vi "__GetDSA_35670A.vi"(11 "DSA_mes":T1={"GPIB_DSA"="11", "Startfrq(Hz)"=0.0, "Stopfrq(Hz)"=800.0, "Range(Vpk)"=1.0, "average"=4}) -> (0 "電圧":dbl[](array[numeric]), 3 "時間":dbl[](array[numeric]))   [LabVIEW 2017]
uses:
  <vilib>/express/express arith-compare/Formula/XNode/ExpressFormulaBlockNode.xnode
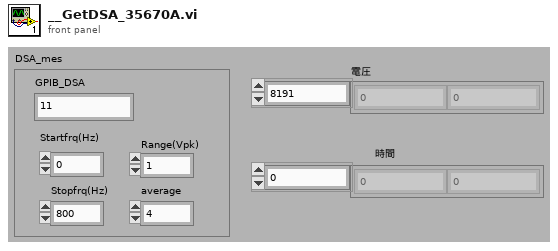
[diagram p1: front panel]
types:
  T1 = cluster{"GPIB_DSA":string, "Startfrq(Hz)":dbl, "Stopfrq(Hz)":dbl, "Range(Vpk)":dbl, "average":i16}
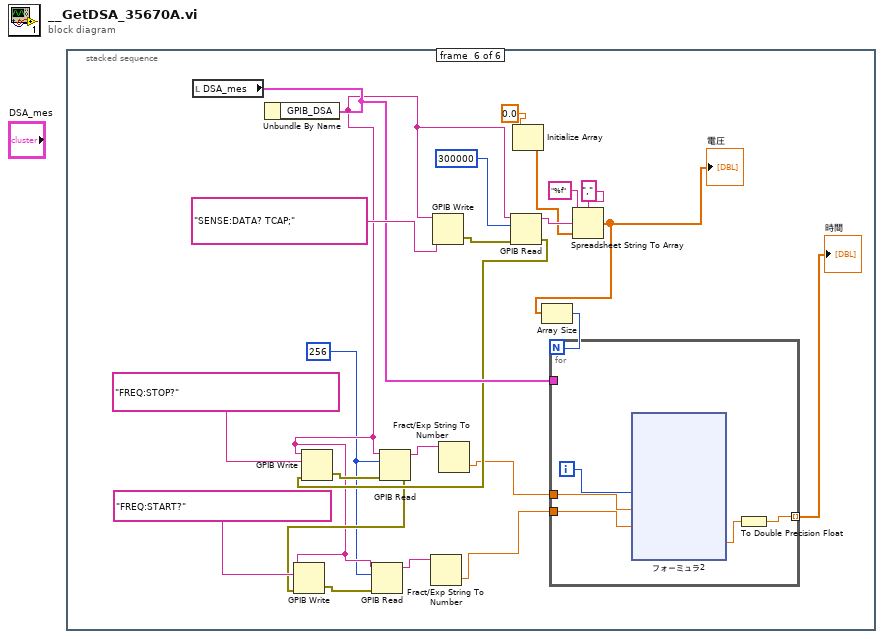
[diagram p0: block diagram]
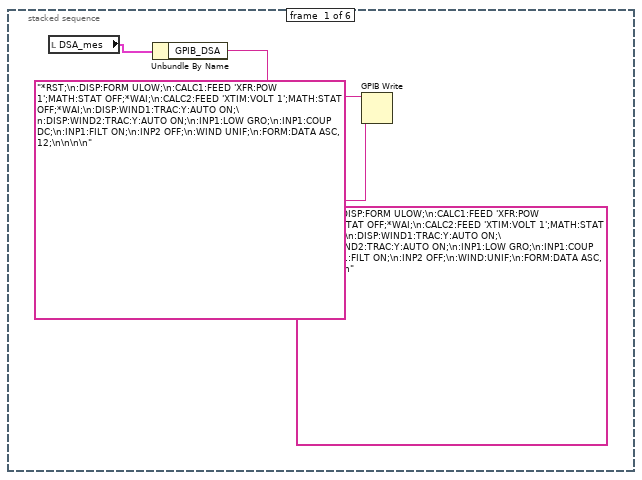
[diagram p2: hidden frame]
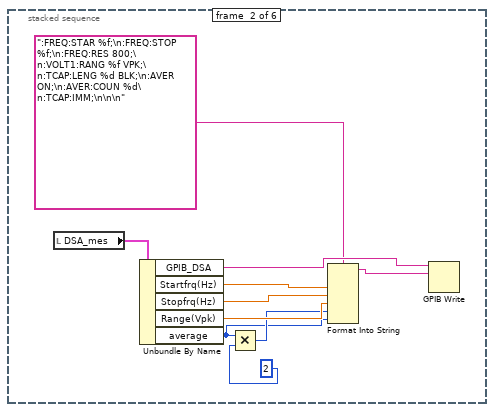
[diagram p3: hidden frame]
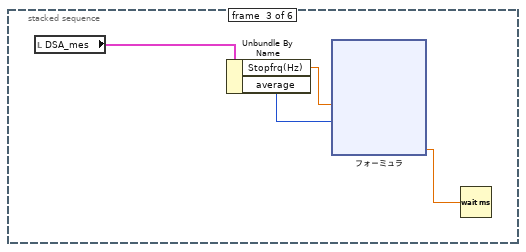
[diagram p4: hidden frame]
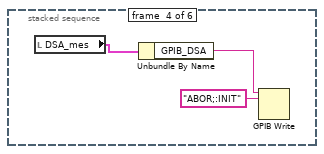
[diagram p5: hidden frame]
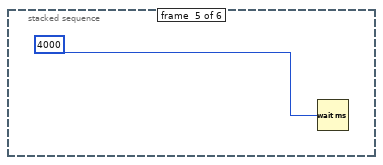
[diagram p6: hidden frame]
diagram:
  n1 = stacked-sequence {
    frame #0 {
      (unwired) "*RST;\n:DISP:FORM ULOW;\n:CALC1:FEED 'XFR:POW 1';MATH:STAT OFF;*WAI;\n:CALC2:FEED 'XTIM:VOLT 1';MATH:STAT OFF;*WAI;\n:DISP:WIND1:TRAC:Y:AUTO ON;\n:DISP:WIND2:TRAC:Y:AUTO ON;\n:INP1:LOW GRO;\n:INP1:COUP DC;\n:INP1:FILT ON;\n:INP2 OFF;\n:WIND:UNIF;\n:FORM:DATA ASC, 12;\n\n\n\n"
      n2 = local read "DSA_mes"() -> (w3:T1)
      n3 = Unbundle By Name(w3) -> ("GPIB_DSA"=w2:string)
      n4 = GPIB Write(0:w2, 1:"*RST;\n:DISP:FORM ULOW;\n:CALC1:FEED 'XFR:POW 1';MATH:STAT OFF;*WAI;\n:CALC2:FEED 'XTIM:VOLT 1';MATH:STAT OFF;*WAI;\n:DISP:WIND1:TRAC:Y:AUTO ON;\n:DISP:WIND2:TRAC:Y:AUTO ON;\n:INP1:LOW GRO;\n:INP1:COUP DC;\n:INP1:FILT ON;\n:INP2 OFF;\n:WIND UNIF;\n:FORM:DATA ASC, 12;\n\n\n\n") -> ()  [unwired: 3 in, 2 out]
    }
    frame #1 {
      n5 = local read "DSA_mes"() -> (w13:T1)
      n6 = Unbundle By Name(w13) -> ("GPIB_DSA"=w12:string, "Startfrq(Hz)"=w10:dbl, "Stopfrq(Hz)"=w9:dbl, "Range(Vpk)"=w7:dbl, "average"=w4:i16)
      n7 = Multiply(x=w4, y=2) -> (x*y=w6:i32)
      n8 = Format Into String(format string=":FREQ:STAR %f;\n:FREQ:STOP %f;\n:FREQ:RES 800;\n:VOLT1:RANG %f VPK;\n:TCAP:LENG %d BLK;\n:AVER ON;\n:AVER:COUN %d\n:TCAP:IMM;\n\n\n", w10, w9, w7, w6, w4) -> (resulting string=w8:string)  [unwired: 2 in, 1 out]
      n9 = GPIB Write(0:w12, 1:w8) -> ()  [unwired: 3 in, 2 out]
    }
    frame #2 {
      n10 = local read "DSA_mes"() -> (w17:T1)
      n11 = Unbundle By Name(w17) -> ("Stopfrq(Hz)"=w16:dbl, "average"=w15:i16)
      n12 = xnode "フォーミュラ"("stop"=w16, "block"=w15) -> ("結果"=w14:dbl)  [unwired: 1 in, 1 out]
      n13 = Wait (ms)(milliseconds to wait=w14) -> ()  [unwired: 1 out]
    }
    frame #3 {
      n14 = local read "DSA_mes"() -> (w30:T1)
      n15 = Unbundle By Name(w30) -> ("GPIB_DSA"=w29:string)
      n16 = GPIB Write(0:w29, 1:"ABOR;:INIT") -> ()  [unwired: 3 in, 2 out]
    }
    frame #4 {
      n17 = Wait (ms)(milliseconds to wait=4000) -> ()  [unwired: 1 out]
    }
    frame #5 {
      w34 = 256
      n18 = local read "DSA_mes"() -> (w46:T1)
      n19 = Unbundle By Name(w46) -> ("GPIB_DSA"=w35:string)
      n20 = GPIB Write(0:w35, 1:"SENSE:DATA? TCAP;") -> (6:w55:errorcluster)  [unwired: 3 in, 1 out]
      n21 = GPIB Read(0:w35, 1:300000, 3:w55) -> (5:w53:string, 7:w42:errorcluster)  [unwired: 2 in, 1 out]
      n22 = GPIB Write(0:w35, 1:"FREQ:STOP?", 3:w42) -> (6:w43:errorcluster)  [unwired: 2 in, 1 out]
      n23 = GPIB Read(0:w35, 1:w34, 3:w43) -> (5:w40:string, 7:w36:errorcluster)  [unwired: 2 in, 1 out]
      n24 = GPIB Write(0:w35, 1:"FREQ:START?", 3:w36) -> (6:w39:errorcluster)  [unwired: 2 in, 1 out]
      n25 = GPIB Read(0:w35, 1:w34, 3:w39) -> (5:w37:string)  [unwired: 2 in, 2 out]
      n26 = Fract/Exp String To Number(string=w37) -> (number=w32:dbl)  [unwired: 3 in, 1 out]
      n27 = Fract/Exp String To Number(string=w40) -> (number=w33:dbl)  [unwired: 3 in, 1 out]
      n28 = Initialize Array(0.0) -> (w48:dbl[])  [unwired: 1 in]
      n29 = Spreadsheet String To Array(delimiter (Tab)=",", format string="%f", spreadsheet string=w53, array type (2D Dbl)=w48) -> (array=w44:dbl[])
      "電圧" <- w44
      n30 = Array Size(array=w44) -> (size(s)=w47:i32)
      n31 = for {
        N: w47 -> [_]
        tunnel: w46 -> [_]
        tunnel: [w58] -> w45 mode=indexing
        tunnel: w33 -> [w57]
        tunnel: w32 -> [w56]
        i -> [w60]
        n32 = xnode "フォーミュラ2"("i"=w60, "stop"=w57, "start"=w56) -> ("結果"=w59:dbl)  [unwired: 1 in, 1 out]
        n33 = To Double Precision Float(number=w59) -> (double precision float=w58:dbl)
      }
      "時間" <- w45
    }
  }
